vi "Front Panel.vi"(11 "GUI In":refnum<class "Pcal GUI.lvclass">) -> ()   [LabVIEW 2015, in "Pcal GUI.lvclass"]
uses:
  Pcal GUI.lvclass
  Reusable/Xctls/Buffer/1D Control/1D Buffer.xctl
  Reusable/GUI/GUI.lvclass/GUI.ctl
  Reusable/Observer/Observer.lvclass/Observer.ctl
  Controls/MFC Address.ctl
  Pcal GUI.lvclass/Pcal GUI.ctl
  Data/cPAS Data.lvclass
  Reusable/Sequence/SEQ/SEQ.lvclass
  Sequence/Pressure Calibration/Builder/P Cal Builder.lvclass
  Sequence/Pressure Calibration/Builder/P Cal Builder.lvclass/P Cal Builder.ctl
  Sequence/Pressure Calibration/Builder/Accessors/Write Pressure.vi
  Sequence/Pressure Calibration/Builder/Accessors/Write Time.vi
  Sequence/Pressure Calibration/Builder/Accessors/Write WaitAtMin.vi
  Accessors/Read Calibrate.vi
  Reusable/GUI/Accessors/Read RegEvent.vi
  Reusable/Observer/Read Data Queue.vi
  Reusable/Data/Data.lvclass
panel:
  in  "Clear":bool
  in  "dTime":dbl=90.0 caption="Dwell Time"
  in  "numSteps":sgl=5.0 caption="Num of Steps"
  out "seqMsg":string[](array[string]) caption="Messages"
  out "P":sgl caption="Pressure (mb)"
  in  "useCurrP":bool=TRUE caption="Initial Pressure Source"
  out "timestamp":timestamp format="%<%H:%M:%S%2u>T"
  out "Alarms":cluster{"Temperature":bool, "Laser RMS":bool}
  in  "Checklist":cluster{"check 1":bool, "check 2":bool}
  in  "psp":sgl caption="Pressure\nSetpoint (mb)"
  out "pPlot":cluster{"time":timestamp, "data":sgl[]}(xcontrol) caption="Pressure Out"
  in  "runCal":bool
  in  "Pressure (mb)":cluster{"Initial":dbl, "Final":dbl}={"Initial"=1000.0, "Final"=400.0}
  # "Pressure Calibration Input"
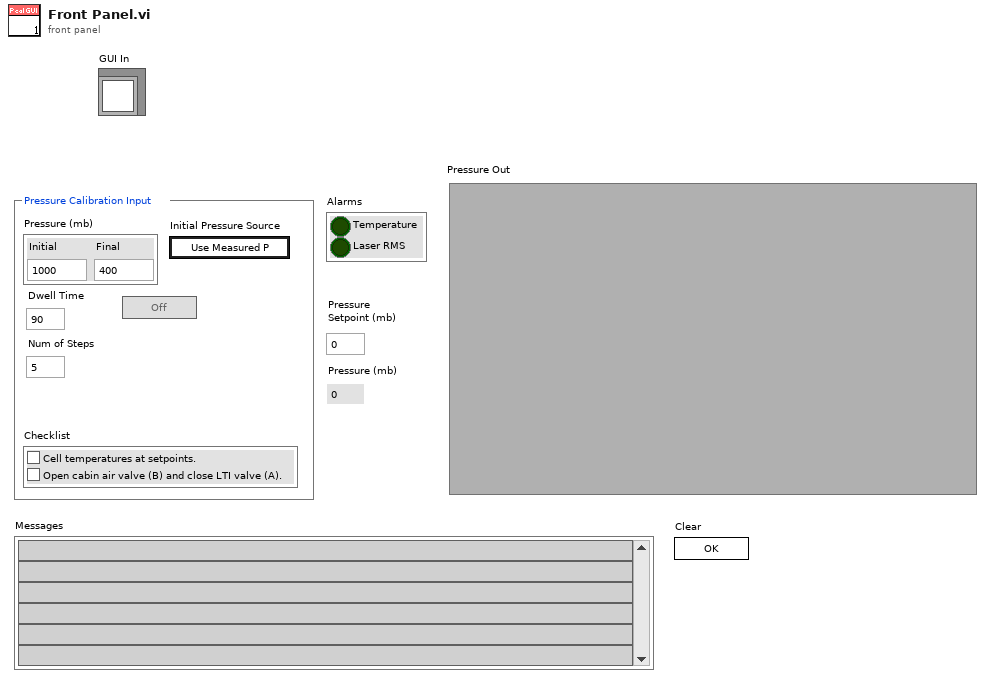
[diagram p1: front panel]
types:
  T1 = enum8{"Enabled", "Disabled", "Disabled and Grayed Out"}
  T2 = cluster{"Name":string, "Line Width":u8, "Line Style":u8, "Color":u32}[]
  T3 = typedef "MFC Address.ctl" = enum16{"CRDS Purge", "CRDS Thermodenuded", "CRDS Dry", "CRDS Med RH", "CRDS High RH", "PAS Ch 1", "PAS Ch 2", "PAS Ch3", "PAS Ch 4", "PAS Ch 5", "CLAP", "O3", "Pinlet"}
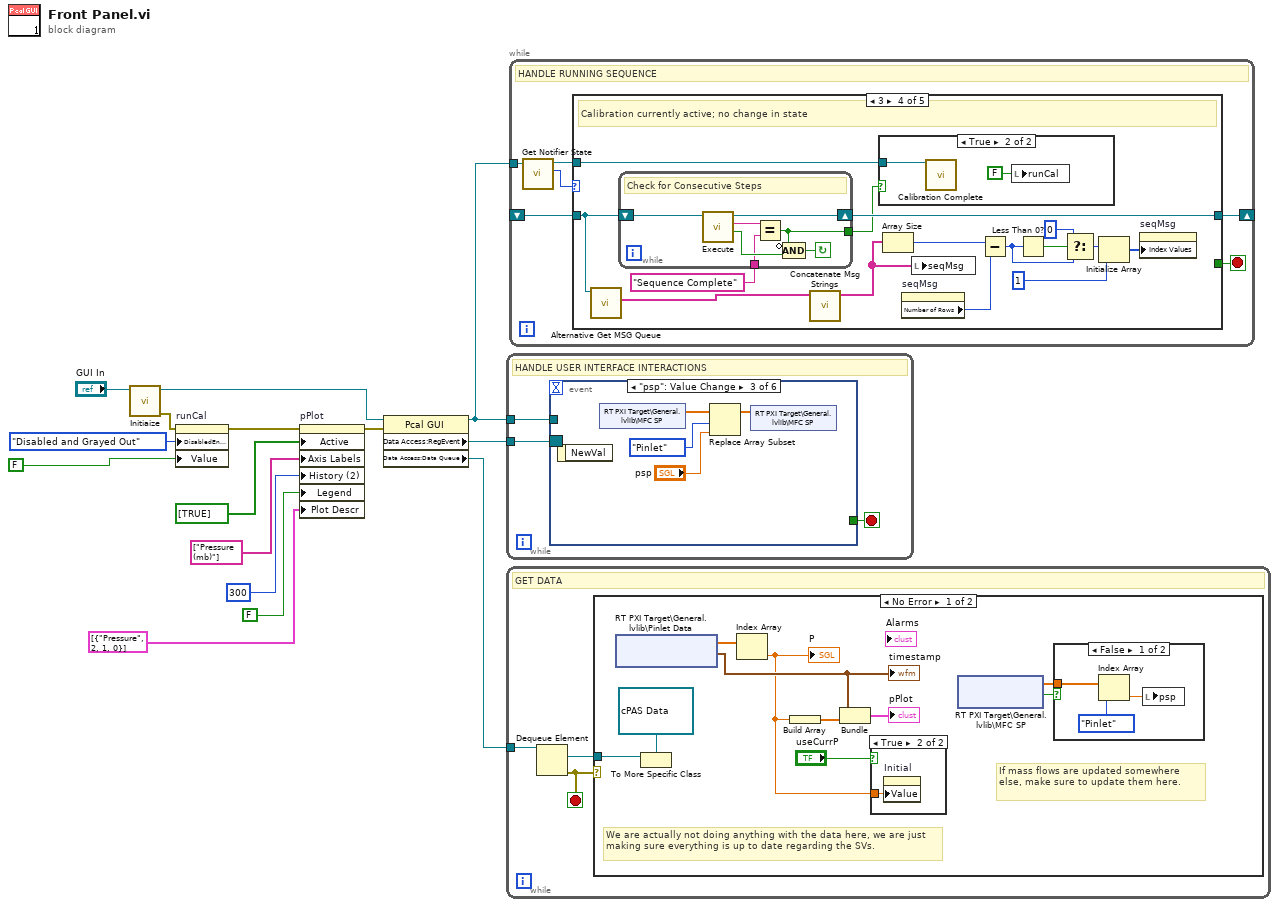
[diagram p0: block diagram]
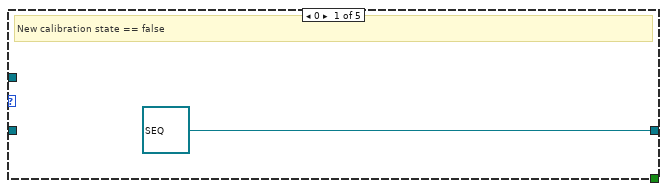
[diagram p2: hidden frame]
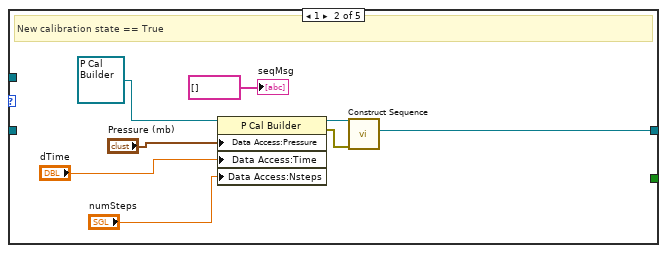
[diagram p3: hidden frame]
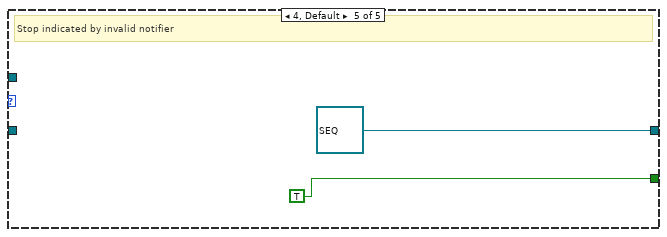
[diagram p6: hidden frame]
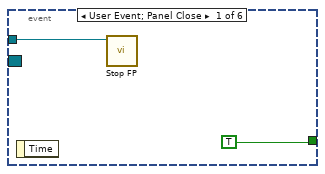
[diagram p10: hidden frame]
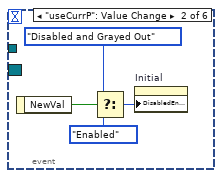
[diagram p11: hidden frame]
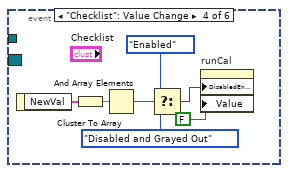
[diagram p12: hidden frame]
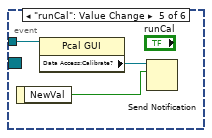
[diagram p13: hidden frame]
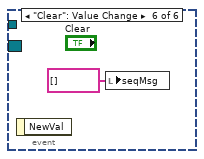
[diagram p14: hidden frame]
diagram:
  n1 = call "Initiaize.vi"("Pcal GUI in"="GUI In") -> ("error out"=w1:errorcluster, "Pcal GUI out"=w2:refnum<class "Pcal GUI.lvclass">)  [unwired: 9 in]
  n2 = property on="runCal" class="Bool (strict)"(error in=w1, "DisabledEnum"=T1."Disabled and Grayed Out" ("Disabled"), "Value"=FALSE ("runCal")) -> (error out=w5:errorcluster)  [unwired: 1 in, 1 out]
  n3 = property on="pPlot" class="1D Buffer (strict)"(error in=w5, "Active"=bool[] [TRUE], "Axis Labels"=string[] ["Pressure (mb)"], "History (2)"=u16 300 ("History"), "Legend"=FALSE, "Plot Descr"=T2 [{"Name"="Pressure", "Line Width"=2, "Line Style"=1, "Color"=0}]) -> (error out=w8:errorcluster)  [unwired: 1 in, 1 out]
  n4 = property class="Pcal GUI"(reference=w2, error in=w8) -> (reference out=w4:refnum<class "Pcal GUI.lvclass">, "Data Access:RegEvent"=w10:refnum<event-registration>, "Data Access:Data Queue"=w9:refnum<queue>)  [unwired: 1 out]
  n5 = while {
    tunnel: w10 -> [w18]
    tunnel: w4 -> [w16]
    stop <- w17 stop-if-true
    # "HANDLE USER INTERFACE INTERACTIONS"
    n6 = event shown="[2] \"psp\": Value Change" {
      selector: w18 -> [_ _ _ _ _ _]
      dyn-events: _ -> [_ _ _ _ _ _]
      timeout: _ -> [_ _ _ _ _ _]
      tunnel: [TRUE _ _ _ _ _] -> w17
      tunnel: w16 -> [w19 _ _ _ w38 _]
      event User Event; Panel Close {
        n7 = event-data() -> ()  [unwired: 1 in, 1 out]
        n8 = call-dynamic "Stop FP.vi"("Pcal GUI in"=w19) -> ()  [unwired: 9 in, 2 out]
      }
      event "useCurrP": Value Change {
        n9 = event-data() -> ("NewVal"=w24:bool)  [unwired: 1 in]
        n10 = Select(t=T1."Disabled and Grayed Out", s=w24, f=T1."Enabled" ("Disabled")) -> (s? t:f=w21:T1)
        n11 = property on="Initial" class="DigNum (strict)"("DisabledEnum"=w21) -> ()  [unwired: 2 in, 2 out]
      }
      event "psp": Value Change {
        n12 = event-data() -> ()  [unwired: 1 in, 1 out]
        n13 = shared-variable "RT PXI Target\\General.lvlib\\MFC SP"() -> (w27:sgl[])  [unwired: 1 in, 1 out]
        n14 = Replace Array Subset(array=w27, new element="psp", index=MFC_Address."Pinlet" ("Controllers")) -> (w28:sgl[])
        n15 = shared-variable "RT PXI Target\\General.lvlib\\MFC SP"(w28) -> ()  [unwired: 1 in, 1 out]
      }
      event "Checklist": Value Change {
        n16 = event-data() -> ("NewVal"=w35:cluster{"check 1":bool, "check 2":bool})  [unwired: 1 in]
        n17 = Cluster To Array(cluster=w35) -> (array=w34:bool[])
        n18 = And Array Elements(Boolean array=w34) -> (logical AND=w33:bool)
        n19 = Select(t=T1."Enabled" ("Disabled"), s=w33, f=T1."Disabled and Grayed Out") -> (s? t:f=w31:T1)
        n20 = property on="runCal" class="Bool (strict)"("DisabledEnum"=w31, "Value"=FALSE ("runCal")) -> ()  [unwired: 2 in, 2 out]
      }
      event "runCal": Value Change {
        n21 = event-data() -> ("NewVal"=w36:bool)  [unwired: 1 in]
        n22 = property class="Pcal GUI"(reference=w38) -> ("Data Access:Calibrate?"=w37:refnum<notifier>)  [unwired: 1 in, 2 out]
        n23 = Send Notification(notification=w36, notifier=w37) -> ()  [unwired: 1 in, 2 out]
      }
      event "Clear": Value Change {
        n24 = event-data() -> ()  [unwired: 1 in, 1 out]
        n25 = local write "seqMsg"(string[] [] ("seqMsg")) -> ()
      }
    }
  }
  n26 = while {
    tunnel: w9 -> [w42]
    stop <- w41 stop-if-true
    # "GET DATA"
    n27 = Dequeue Element(queue=w42) -> (element=w40:refnum<data-value>, error out=w41:errorcluster)  [unwired: 2 in, 2 out]
    n28 = case shown="No Error" w41 {
      tunnel: w40 -> [w51 _]
      frame No Error {
        # "We are actually not doing anything with the data here, we are just making sure everything is up to date regarding the SVs."
        # "If mass flows are updated somewhere else, make sure to update them here."
        n29 = shared-variable "RT PXI Target\\General.lvlib\\Pinlet Data"() -> (w47:sgl[], w49:timestamp)  [unwired: 1 in, 1 out]
        "timestamp" <- w49
        n30 = To More Specific Class(target class=refnum<data-value> refnum ("DVR"), reference=w51) -> ()  [unwired: 1 in, 2 out]
        n31 = Index Array(array=w47) -> (element=w43:sgl)  [unwired: 1 in]
        "P" <- w43
        n32 = Build Array(w43) -> (w48:sgl[])
        n33 = Bundle(w49, w48) -> (→"pPlot":cluster{timestamp, sgl[]})  [unwired: 1 in]
        n34 = case shown="True" "useCurrP" {
          tunnel: w43 -> [_ w56]
          frame False {
          }
          frame True {
            n35 = property on="Initial" class="DigNum (strict)"("Value"=w56) -> ()  [unwired: 2 in, 2 out]
          }
        }
        n36 = shared-variable "RT PXI Target\\General.lvlib\\MFC SP"() -> (w44:sgl[], w45:bool)  [unwired: 2 in, 1 out]
        n37 = case shown="False" w45 {
          tunnel: w44 -> [w55 _]
          frame False {
            n38 = Index Array(array=w55, index=MFC_Address."Pinlet" ("Controllers")) -> (element=w53:sgl)
            n39 = local write "psp"(w53) -> ()
          }
          frame True {
          }
        }
      }
      frame Error {
        # "Data Queue is dead -we are stopping since this is controlled by the stop action."
      }
    }
  }
  n40 = while {
    tunnel: w4 -> [w62]
    shift-right: [w58] -> _
    shift-left: _ -> [w57]
    stop <- w60 stop-if-true
    # "HANDLE RUNNING SEQUENCE"
    n41 = call "Get Notifier State.vi"("Pcal GUI in"=w62) -> ("Action"=w59:u32, "Pcal GUI out"=w61:refnum<class "Pcal GUI.lvclass">)  [unwired: 8 in, 1 out]
    n42 = case shown="3" w59 {
      tunnel: [refnum<class "SEQ.lvclass"> refnum ("New Sequence") w71 w72 w87 refnum<class "SEQ.lvclass"> refnum ("New Sequence")] -> w58
      tunnel: w57 -> [_ _ w72 w85 _]
      tunnel: w61 -> [_ _ _ w86 _]
      tunnel: [_ _ _ _ TRUE] -> w60
      frame 0 {
        # "New calibration state == false"
      }
      frame 1 {
        # "New calibration state == True"
        n43 = property class="P Cal Builder"(reference=refnum<class "P Cal Builder.lvclass"> refnum ("P Cal Builder"), "Data Access:Pressure"="Pressure (mb)", "Data Access:Time"="dTime", "Data Access:Nsteps"="numSteps") -> (reference out=w68:refnum<class "P Cal Builder.lvclass">, error out=w65:errorcluster)  [unwired: 1 in]
        n44 = call-dynamic "Construct Sequence.vi"("error in"=w65, "P Cal Builder in"=w68) -> ("New Sequence"=w71:refnum<class "SEQ.lvclass">)  [unwired: 7 in, 2 out]
        "seqMsg" <- string[] [] ("seqMsg")
      }
      frame 2 {
        # "This case should never execute as the wait time should be -1"
      }
      frame 3 {
        # "Calibration currently active; no change in state"
        n45 = call "Alternative Get MSG Queue.vi"("SEQ in"=w85) -> ("seqMsg"=w82:string[])  [unwired: 8 in, 2 out]
        n46 = while {
          shift-right: [w93] -> w87
          shift-left: w85 -> [w94]
          tunnel: [w90] -> w84
          tunnel: "Sequence Complete" ("t") -> [w88]
          stop <- w91 continue-if-true
          # "Check for Consecutive Steps"
          n47 = call-dynamic "Execute.vi"("SEQ in"=w94) -> ("Next Step?"=w89:bool, "MSG"=w92:string, "SEQ out"=w93:refnum<class "SEQ.lvclass">)  [unwired: 7 in, 1 out]
          n48 = Equal?(x=w92, y=w88) -> (x = y?=w90:bool)
          n49 = Compound Arithmetic op=AND(invert w90, w89) -> (w91:bool)
        }
        n50 = call "Concatenate Msg Strings.vi"("StringsIn"=w82) -> ("StringsOut"=w81:string[])  [unwired: 10 in]
        n51 = case shown="True" w84 {
          tunnel: w86 -> [_ w96]
          frame False {
          }
          frame True {
            n52 = call "Calibration Complete.vi"("Pcal GUI in"=w96) -> ()  [unwired: 9 in, 2 out]
            n53 = local write "runCal"(FALSE ("runCal")) -> ()
          }
        }
        n54 = Array Size(array=w81) -> (size(s)=w75:i32)
        n55 = property on="seqMsg" class="Arr (strict)"() -> ("Number of Rows"=w74:u32)  [unwired: 2 in, 2 out]
        n56 = local write "seqMsg"(w81) -> ()
        n57 = Subtract(x=w75, y=w74) -> (x-y=w78:u32)
        n58 = Less Than 0?(x=w78) -> (x < 0?=w77:bool)
        n59 = Select(t=u32 0, s=w77, f=w78) -> (s? t:f=w80:u32)
        n60 = Initialize Array(w80, 1 ("dimension size")) -> (w73:u32[])
        n61 = property on="seqMsg" class="Arr (strict)"("Index Values"=w73) -> ()  [unwired: 2 in, 2 out]
      }
      frame 4, Default {
        # "Stop indicated by invalid notifier"
      }
    }
  }
